vi "Bump Turret Az.vi"(8 "reset":bool, 9 "D":dbl, 10 "d":dbl, 11 "D-Pad":dbl) -> (3 "offset":dbl)   [LabVIEW 2016]
panel:
  out "arctan(x)":dbl
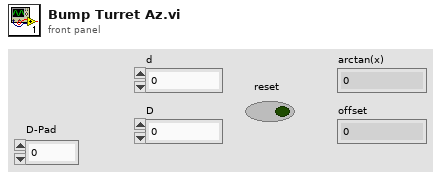
[diagram p1: front panel]
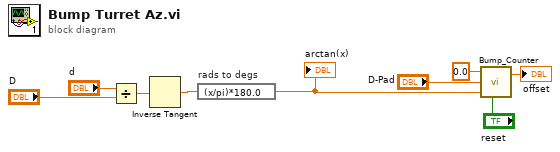
[diagram p0: block diagram]
diagram:
  n1 = Divide(x="d", y="D") -> (x/y=w8:dbl)
  n2 = Inverse Tangent(1:w8) -> (0:w7:dbl)
  n3 = expression code="(x/pi)*180.0" "rads to degs"(w7) -> (w4:dbl)
  "arctan(x)" <- w4
  n4 = call <userlib>:"Bump_Counter.vi"("ref"=0.0, "cntrl"="D-Pad", "quanta"=w4, "reset"="reset") -> ("out"=→"offset":dbl)  [unwired: 2 in]
